vi "Model_Test.vi"() -> ()   [LabVIEW 2019]
panel:
  in  "Disturbance":dbl=5.0
  in  "Load Setpoint":dbl=20.0 format="%#_13g"
  out "Simulated Load":dbl
  in  "stop":bool
  out "Simulated Position":dbl(graph)
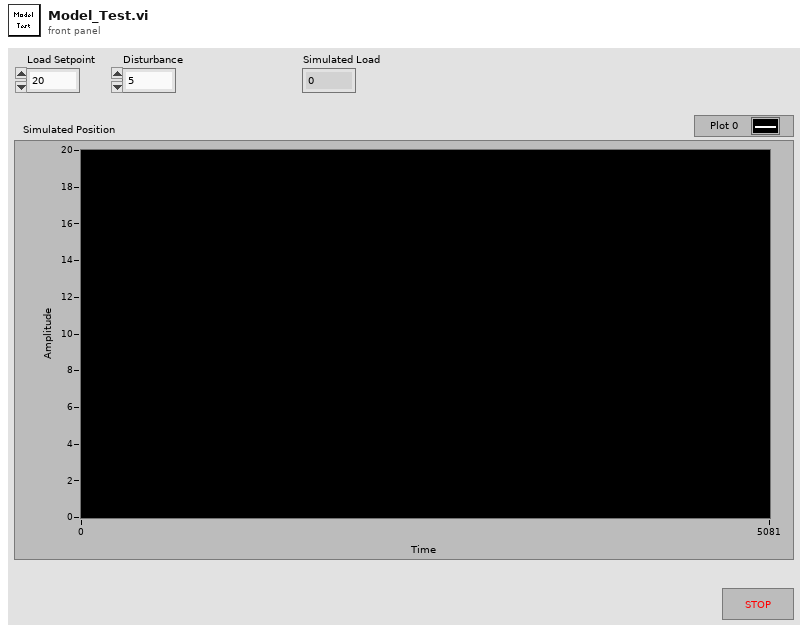
[diagram p1: front panel]
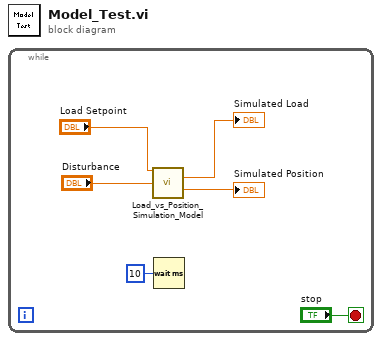
[diagram p0: block diagram]
diagram:
  n1 = while {
    stop <- "stop" stop-if-true
    n2 = call "Load_vs_Position_Simulation_Model.vi"("Load Setpoint"="Load Setpoint", "Disturbance"="Disturbance") -> ("Simulated Load"=→"Simulated Load":dbl, "Simulated Position"=→"Simulated Position":dbl)  [unwired: 12 in]
    n3 = Wait (ms)(milliseconds to wait=u32 10) -> ()  [unwired: 1 out]
  }
